vi "svl_Max-Min Resampled Level (1 Ch).vi"(8 "error in (no error)":errorcluster, 9 "processing state":T1(ring), 11 "scaled even angle signal":T2 {"even angle signal" format="%.2f"; "dr" format="%.2f"; "r0" format="%.2f"}) -> (0 "error out":errorcluster, 1 "max-min level":dbl format="%.2f", 2 "final min level":dbl format="%.2f", 3 "final max level":dbl format="%.2f")   [LabVIEW 2017]
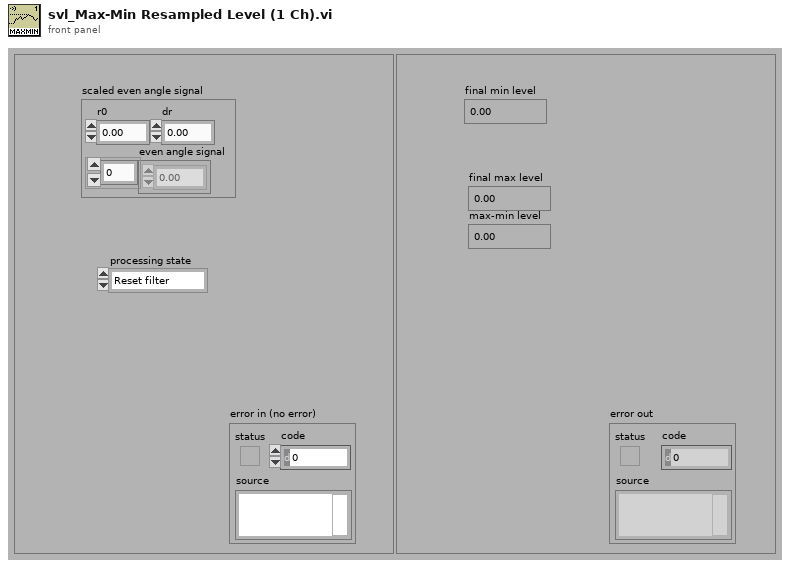
[diagram p1: front panel]
types:
  T1 = enum16{"Reset filter", "Restart averaging", "Continue processing"}
  T2 = cluster{"r0":dbl, "dr":dbl, "even angle signal":dbl[]}
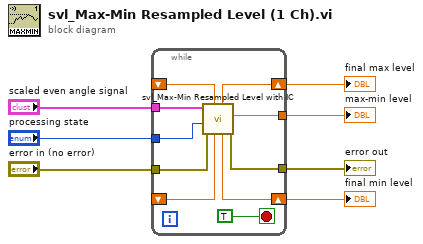
[diagram p0: block diagram]
diagram:
  n1 = while {
    tunnel: [w15] -> w4
    tunnel: "error in (no error)" -> [w16]
    tunnel: "processing state" -> [w12]
    tunnel: "scaled even angle signal" -> [w17]
    shift-right: [w10] -> w1
    shift-left: _ -> [w11]
    shift-right: [w8] -> w2
    shift-left: _ -> [w9]
    tunnel: [w13] -> w3
    stop <- TRUE stop-if-true
    n2 = call <vilib>:"svl_Max-Min Resampled Level with IC.vi"("initial min level"=w9, "initial max level"=w11, "error in (no error)"=w16, "processing state"=w12, "even angle signal"=w17) -> ("error out"=w15:errorcluster, "max-min level"=w13:dbl, "final min level"=w8:dbl, "final max level"=w10:dbl)  [unwired: 3 in]
  }
  "final min level" <- w2
  "error out" <- w4
  "max-min level" <- w3
  "final max level" <- w1
